vi "Player Info.vi"(11 "Team 3 in":refnum<class "Team 3.lvclass">) -> (0 "Defeat Speech":string, 1 "Victory Speech":string, 2 "Name":string, 3 "Team 3 out":refnum<class "Team 3.lvclass">)   [LabVIEW 2015, in "Team 3.lvclass"]
uses:
  Team 3.lvclass
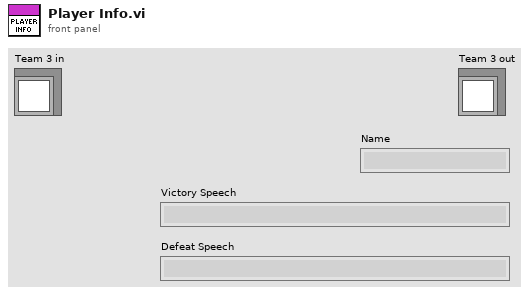
[diagram p1: front panel]
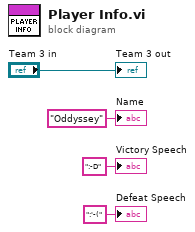
[diagram p0: block diagram]
diagram:
  "Team 3 out" <- "Team 3 in"
  "Name" <- "Oddyssey" ("Name")
  "Victory Speech" <- ":-D" ("Victory Speech")
  "Defeat Speech" <- ":'-(" ("Defeat Speech")
